vi "BINHDR_P_write.vi"(8 "error in (no error)":errorcluster, 10 "BINHDR_P":T1, 11 "refnum in":refnum<file>) -> (0 "error out":errorcluster, 3 "refnum out":refnum<file>)   [LabVIEW 2012]
uses:
  TTTR_data_headers/BINHDR_P.ctl
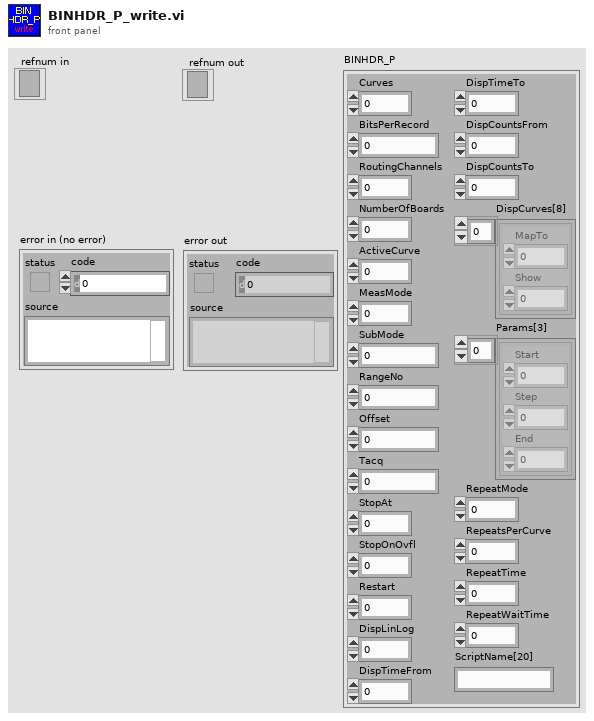
[diagram p1: front panel]
types:
  T1 = typedef "BINHDR_P.ctl" = cluster{"Curves":i32, "BitsPerRecord":i32, "RoutingChannels":i32, "NumberOfBoards":i32, "ActiveCurve":i32, "MeasMode":i32, "SubMode":i32, "RangeNo":i32, "Offset":i32, "Tacq":i32, "StopAt":i32, "StopOnOvfl":i32, "Restart":i32, "DispLinLog":i32, "DispTimeFrom":i32, "DispTimeTo":i32, "DispCountsFrom":i32, "DispCountsTo":i32, "DispCurves[8]":cluster{"MapTo":i32, "Show":i32}[], "Params[3]":cluster{"Start":sgl, "Step":sgl, "End":sgl}[], "RepeatMode":i32, "RepeatsPerCurve":i32, "RepeatTime":i32, "RepeatWaitTime":i32, "ScriptName[20]":string}
  T2 = enum16{"big-endian, network order", "native, host order", "little-endian"}
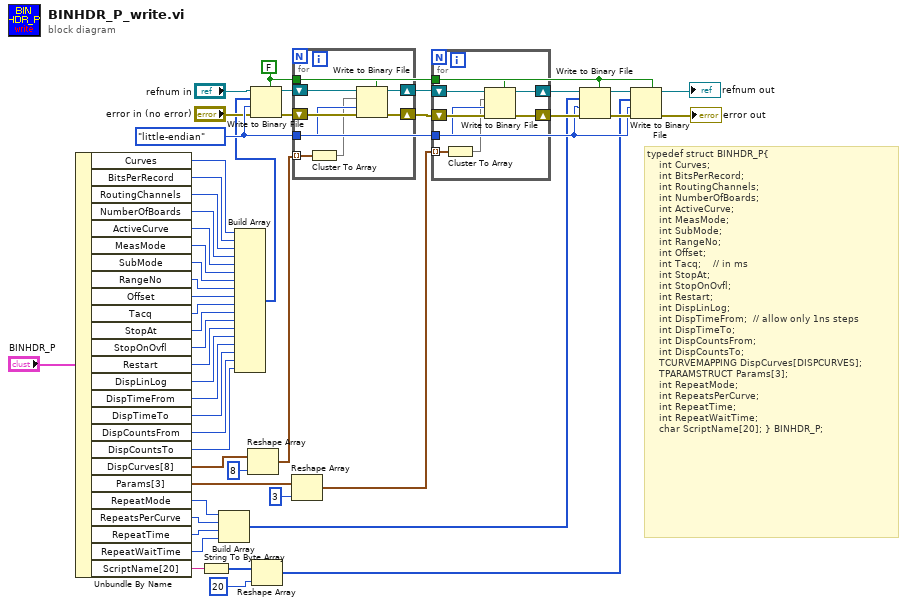
[diagram p0: block diagram]
diagram:
  w8 = FALSE ("prepend array or string size? (T)")
  w39 = T2."little-endian" ("byte order (0:big-endian, network order)")
  # "typedef struct BINHDR_P{\n\t\t\t\tint Curves;\n\t\t\t\tint BitsPerRecord;\n\t\t\t\tint RoutingChannels;\n\t\t\t\tint NumberOfBoards;\n\t\t\t\tint ActiveCurve;\n\t\t\t\tint MeasMode;\n\t\t\t\tint SubMode;\n\t\t\t\tint RangeNo;\n\t\t\t\tint Offset;\n\t\t\t\tint Tacq;\t\t\t\t// in ms\n\t\t\t\tint StopAt;\n\t\t\t\tint StopOnOvfl;\n\t\t\t\tint Restart;\n\t\t\t\tint DispLinLog;\n\t\t\t\tint DispTimeFrom;\t\t// allow only 1ns steps\n\t\t\t\tint DispTimeTo;\n\t\t\t\tint DispCountsFrom;\n\t\t\t\tint DispCountsTo;\n\t\t\t\tTCURVEMAPPING DispCurves[DISPCURVES];\t\n\t\t\t\tTPARAMSTRUCT Params[3];\n\t\t\t\tint RepeatMode;\n\t\t\t\tint RepeatsPerCurve;\n\t\t\t\tint RepeatTime;\n\t\t\t\tint RepeatWaitTime;\n\t\t\t\tchar ScriptName[20];\t} BINHDR_P;"
  n1 = Unbundle By Name("BINHDR_P") -> ("Curves"=w35:i32, "BitsPerRecord"=w34:i32, "RoutingChannels"=w33:i32, "NumberOfBoards"=w32:i32, "ActiveCurve"=w31:i32, "MeasMode"=w30:i32, "SubMode"=w29:i32, "RangeNo"=w28:i32, "Offset"=w27:i32, "Tacq"=w26:i32, "StopAt"=w25:i32, "StopOnOvfl"=w24:i32, "Restart"=w23:i32, "DispLinLog"=w22:i32, "DispTimeFrom"=w21:i32, "DispTimeTo"=w20:i32, "DispCountsFrom"=w19:i32, "DispCountsTo"=w18:i32, "DispCurves[8]"=w6:cluster{"MapTo":i32, "Show":i32}[], "Params[3]"=w3:cluster{"Start":sgl, "Step":sgl, "End":sgl}[], "RepeatMode"=w12:i32, "RepeatsPerCurve"=w13:i32, "RepeatTime"=w14:i32, "RepeatWaitTime"=w15:i32, "ScriptName[20]"=w16:string)
  n2 = String To Byte Array(string=w16) -> (unsigned byte array=w11:u8[])
  n3 = Build Array(w12, w13, w14, w15) -> (w7:i32[])
  n4 = Build Array(w35, w34, w33, w32, w31, w30, w29, w28, w27, w26, w25, w24, w23, w22, w21, w20, w19, w18) -> (w17:i32[])
  n5 = Reshape Array(w6, 8) -> (w4:cluster{"MapTo":i32, "Show":i32}[])
  n6 = Write to Binary File(file (use dialog)="refnum in", data=w17, error in="error in (no error)", 5:w8, 9:w39) -> (refnum out=w48:refnum<file>, error out=w49:errorcluster)  [unwired: 1 in, 1 out]
  n7 = Reshape Array(w11, 20 ("count (1)")) -> (w9:u8[])
  n8 = Reshape Array(w3, 3) -> (w1:cluster{"Start":sgl, "Step":sgl, "End":sgl}[])
  n9 = for {
    shift-right: [w54] -> w46
    shift-left: w49 -> [w57]
    shift-right: [w55] -> w47
    shift-left: w48 -> [w56]
    tunnel: w39 -> [w53]
    tunnel: w8 -> [w52]
    tunnel: w4 -> [w51] mode=indexing
    n10 = Cluster To Array(cluster=w51) -> (array=w50:i32[])
    n11 = Write to Binary File(file (use dialog)=w56, data=w50, error in=w57, 5:w52, 9:w53) -> (refnum out=w55:refnum<file>, error out=w54:errorcluster)  [unwired: 1 in, 1 out]
  }
  n12 = for {
    shift-right: [w63] -> w44
    shift-left: w46 -> [w65]
    shift-right: [w62] -> w45
    shift-left: w47 -> [w64]
    tunnel: w39 -> [w61]
    tunnel: w8 -> [w60]
    tunnel: w1 -> [w59] mode=indexing
    n13 = Cluster To Array(cluster=w59) -> (array=w58:sgl[])
    n14 = Write to Binary File(file (use dialog)=w64, data=w58, error in=w65, 5:w60, 9:w61) -> (refnum out=w62:refnum<file>, error out=w63:errorcluster)  [unwired: 1 in, 1 out]
  }
  n15 = Write to Binary File(file (use dialog)=w45, data=w7, error in=w44, 5:w8, 9:w39) -> (refnum out=w42:refnum<file>, error out=w43:errorcluster)  [unwired: 1 in, 1 out]
  n16 = Write to Binary File(file (use dialog)=w42, data=w9, error in=w43, 5:w8, 9:w39) -> (refnum out=→"refnum out":refnum<file>, error out=→"error out":errorcluster)  [unwired: 1 in, 1 out]
